vi "LJU3_init.vi"(7 "Address":string="0", 8 "error in":errorcluster, 11 "channel_list":i32[](array[numeric])) -> (0 "error out":errorcluster, 3 "handle":i32, 4 "status":bool, 5 "mode_list":string[](array[string]))   [LabVIEW 2019]
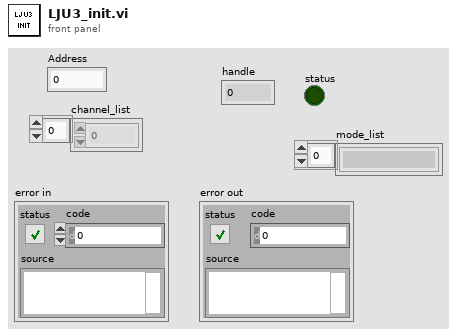
[diagram p1: front panel]
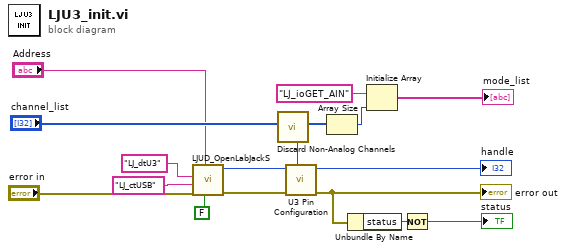
[diagram p0: block diagram]
diagram:
  n1 = call "LJUD_OpenLabJackS.vi"("FirstFound"=FALSE, "Address"="Address", "error in"="error in", "ConnectionType"="LJ_ctUSB", "DeviceType"="LJ_dtU3") -> ("error out"=w12:errorcluster, "Handle"=w14:i32)  [unwired: 4 in, 1 out]
  n2 = call "Discard Non-Analog Channels.vi"("Channels In"="channel_list") -> ("Channels Out"=w4:i32[], "FIO/EIO Analog Enable"=w16:i32)  [unwired: 7 in, 2 out]
  n3 = call "U3 Pin Configuration.vi"("FIO/EIO Analog Enable"=w16, "error in"=w12, "Handle In"=w14) -> ("error out"=w3:errorcluster, "Handle Out"=→"handle":i32)  [unwired: 7 in]
  "error out" <- w3
  n4 = Array Size(array=w4) -> (size(s)=w15:i32)
  n5 = Unbundle By Name(w3) -> ("status"=w2:bool)
  n6 = Initialize Array("LJ_ioGET_AIN" ("IOType"), w15) -> (→"mode_list":string[])
  n7 = Not(x=w2) -> (.not. x?=→"status":bool)
